vi "SUB InstPhase_Wavelet.vi"(9 "Bandwidth":cluster{"frequency":dbl, "+- f":dbl}={"frequency"=444.0, "+- f"=50.0}, 10 "scale info":variant, 11 "scalogram matrix":cdb[][](array[numeric])) -> (2 "Delta_IP":waveform(dbl), 3 "IA":waveform(dbl))   [LabVIEW 2017]
uses:
  <vilib>/Analysis/NI_AALPro.lvlib
  <vilib>/addons/_Advanced Signal Processing/NI_AdvSigProcWA.lvlib
panel:
  out "dt":dbl
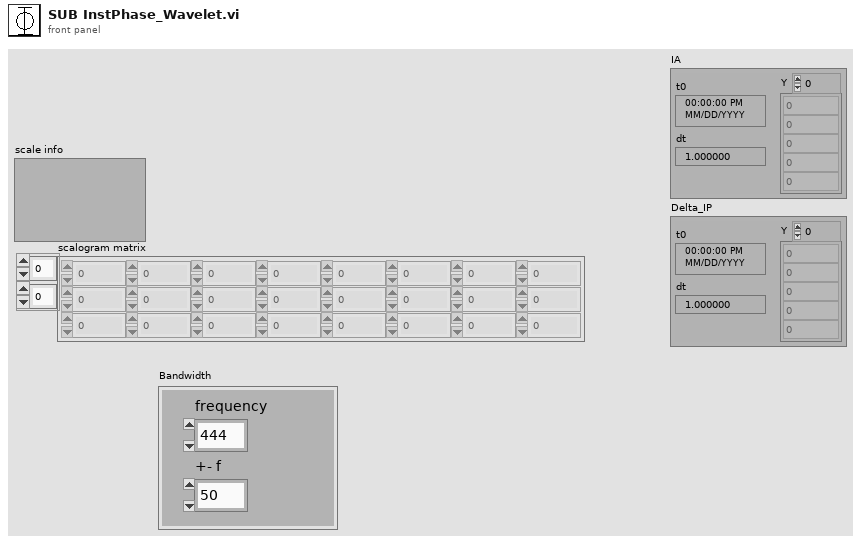
[diagram p1: front panel]
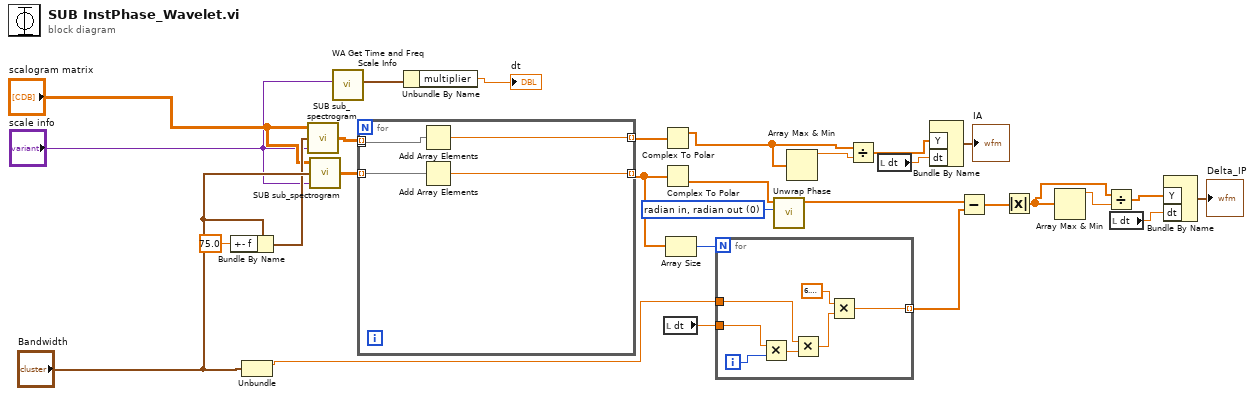
[diagram p0: block diagram]
diagram:
  w15 = 0 items=["radian in, radian out", "radian in, degree out", "degree in, degree out", "degree in, radian out"] ("phase unit")
  n1 = Bundle By Name(cluster="Bandwidth", "+- f"=75.0) -> (w8:cluster{"frequency":dbl, "+- f":dbl})
  n2 = Unbundle("Bandwidth") -> ("frequency"=w25:dbl)  [unwired: 1 out]
  n3 = call "SUB sub_spectrogram.vi"("scale info"="scale info", "Bandwidth"=w8, "scalogram matrix"="scalogram matrix") -> ("sub_Spectrogram"=w12:cdb[][])
  n4 = call "SUB sub_spectrogram.vi"("scale info"="scale info", "Bandwidth"="Bandwidth", "scalogram matrix"="scalogram matrix") -> ("sub_Spectrogram"=w29:cdb[][])
  n5 = call <vilib>:"WA Get Time and Freq Scale Info.vi"("scale info"="scale info") -> ("time info"=w6:cluster{"offset":dbl, "multiplier":dbl})  [unwired: 1 in, 9 out]
  n6 = for {
    tunnel: w29 -> [w33] mode=indexing
    tunnel: [w32] -> w27 mode=indexing
    tunnel: [w31] -> _ mode=indexing
    tunnel: w12 -> [w31] mode=indexing
    tunnel: [w30] -> w11 mode=indexing
    n7 = Add Array Elements(numeric array=w31) -> (sum=w30:cdb)
    n8 = Add Array Elements(numeric array=w33) -> (sum=w32:cdb)
  }
  n9 = Unbundle By Name(w6) -> ("multiplier"=→"dt":dbl)
  n10 = Complex To Polar(r * e^(i*theta)=w11) -> (r=w10:dbl[])  [unwired: 1 out]
  n11 = Complex To Polar(r * e^(i*theta)=w27) -> (theta=w16:dbl[])  [unwired: 1 out]
  n12 = local read "dt"() -> (w26:dbl)
  n13 = Array Size(array=w27) -> (size(s)=w28:i32)
  n14 = for {
    N: w28 -> [_]
    tunnel: w26 -> [w39]
    tunnel: w25 -> [w37]
    tunnel: [w34] -> w24 mode=indexing
    i -> [w40]
    n15 = Multiply(x=w39, y=w40) -> (x*y=w38:dbl)
    n16 = Multiply(x=w37, y=w38) -> (x*y=w35:dbl)
    n17 = Multiply(x=6.283185307179586, y=w35) -> (x*y=w34:dbl)
  }
  n18 = call <vilib>:"Unwrap Phase.vi"("phase unit"=w15, "Phase"=w16) -> ("Unwrapped Phase"=w13:dbl[])  [unwired: 8 in, 1 out]
  n19 = Array Max & Min(array=w10) -> (max value=w23:dbl)  [unwired: 3 out]
  n20 = Divide(x=w10, y=w23) -> (x/y=w22:dbl[])
  n21 = local read "dt"() -> (w21:dbl)
  n22 = Bundle By Name("Y"=w22, "dt"=w21) -> (→"IA":waveform(dbl))  [unwired: 1 in]
  n23 = Subtract(x=w13, y=w24) -> (x-y=w14:dbl[])
  n24 = Absolute Value(x=w14) -> (abs(x)=w20:dbl[])
  n25 = Array Max & Min(array=w20) -> (max value=w19:dbl)  [unwired: 3 out]
  n26 = Divide(x=w20, y=w19) -> (x/y=w18:dbl[])
  n27 = local read "dt"() -> (w17:dbl)
  n28 = Bundle By Name("Y"=w18, "dt"=w17) -> (→"Delta_IP":waveform(dbl))  [unwired: 1 in]
